vi "NADC Modify Standard.vi"(0 "VISA Resource Name":refnum<visa-resource-name>, 1 "Filter (T:RNYQ)":bool=TRUE, 2 "Filter Alpha (0.35)":dbl=0.35 format="%.2f", 3 "Bit Rate (48.600)":dbl=48.6 format="%.3f", 5 "Phase Polarity (T:NORMAL)":bool=TRUE, 7 "Burst Rise Time (5.860)":dbl=5.86 format="%.3f", 9 "Burst Rise Delay (9.000)":dbl=9.0 format="%.3f", 11 "error in (no error)":errorcluster {"code" format="%.0x"}, 12 "Burst Fall Time (5.470)":dbl=5.47 format="%.3f", 13 "Burst Fall Delay (9.000)":dbl=9.0 format="%.3f") -> (4 "VISA Resource Name Out":refnum<visa-resource-name>, 15 "error out":errorcluster {"code" format="%.0x"})   [LabVIEW 2014, in "Agilent ESG Series.lvlib"]
doc: "This VI is used to configure the \"Modify Standard\" parameters."
uses:
  Agilent ESG Series.lvlib
panel:
  # "NORMAL"
  # "RNYQ"
  # "NYQ"
  # "INVERT"
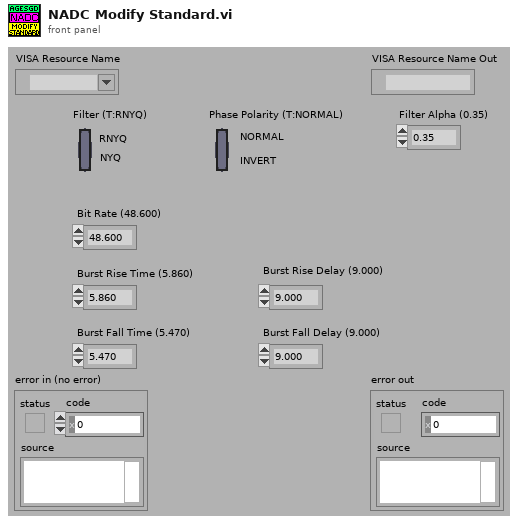
[diagram p1: front panel]
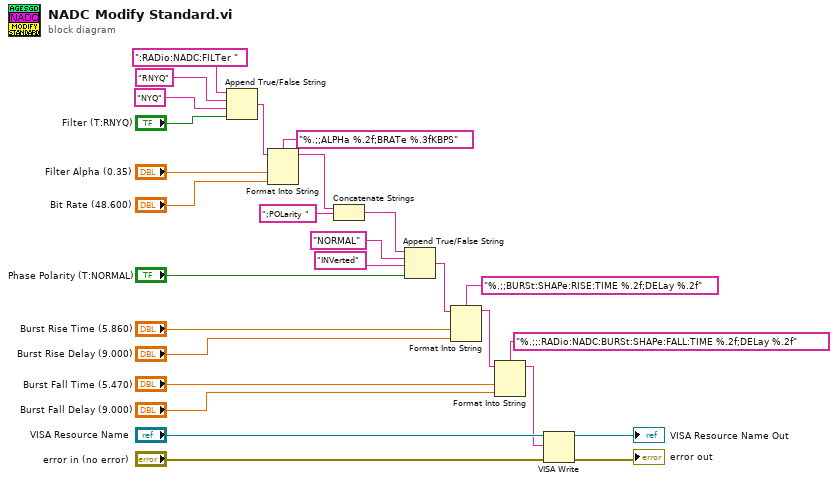
[diagram p0: block diagram]
diagram:
  n1 = Append True/False String(1:"Filter (T:RNYQ)", 2:"NYQ" ("false string"), 3:"RNYQ" ("true string"), 4:":RADio:NADC:FILTer ") -> (0:w13:string)
  n2 = Format Into String(format string="%.;;ALPHa %.2f;BRATe %.3fKBPS", initial string=w13, "Filter Alpha (0.35)", "Bit Rate (48.600)") -> (resulting string=w11:string)  [unwired: 1 in, 1 out]
  n3 = Concatenate Strings(w11, ";POLarity ") -> (w18:string)
  n4 = Append True/False String(1:"Phase Polarity (T:NORMAL)", 2:"INVerted" ("false string"), 3:"NORMAL" ("true string"), 4:w18) -> (0:w9:string)
  n5 = Format Into String(format string="%.;;BURSt:SHAPe:RISE:TIME %.2f;DELay %.2f", initial string=w9, "Burst Rise Time (5.860)", "Burst Rise Delay (9.000)") -> (resulting string=w5:string)  [unwired: 1 in, 1 out]
  n6 = Format Into String(format string="%.;;:RADio:NADC:BURSt:SHAPe:FALL:TIME %.2f;DELay %.2f", initial string=w5, "Burst Fall Time (5.470)", "Burst Fall Delay (9.000)") -> (resulting string=w1:string)  [unwired: 1 in, 1 out]
  n7 = VISA Write(VISA resource name="VISA Resource Name", write buffer=w1, error in (no error)="error in (no error)") -> (VISA resource name out=→"VISA Resource Name Out":refnum<visa-resource-name>, error out=→"error out":errorcluster)  [unwired: 1 out]
